vi "init_chromatic_confocal.vi"(6 "Port":u32, 7 "IP Address":u8[](array[numeric])=[192, 168, 1, 1], 9 "timeout":u32=5000 caption="Timeout", 10 "Device ID":i32 min=0 max=2, 11 "Comm Interface":enum8{"USB", "ETHERNET"}(ring)) -> (0 "error out":errorcluster {"code" format="%x"})   [LabVIEW 2020]
uses:
  Keyence CL-3000/Public/clusters/CL3IF_ETHERNET_SETTING.ctl
  Keyence CL-3000/Keyence CL-3000.lvlib
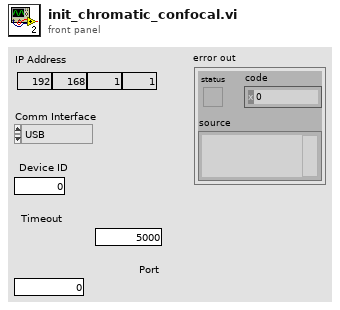
[diagram p1: front panel]
types:
  T1 = typedef "Keyence CL-3000.lvlib/CL3IF_ETHERNET_SETTING.ctl" = cluster{"IP Address":cluster{"IP1":u8, "IP2":u8, "IP3":u8, "IP4":u8}, "portNo":u32}
  T2 = cluster{"IP Address":u8, "IP Address":u8, "IP Address":u8, "IP Address":u8}
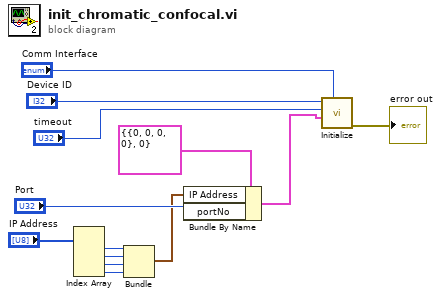
[diagram p0: block diagram]
diagram:
  n1 = Index Array(array="IP Address") -> (element #1=w4:u8, element #2=w5:u8, element #3=w6:u8, element #4=w7:u8)  [unwired: 4 in]
  n2 = Bundle("IP Address"=w4, "IP Address"=w5, "IP Address"=w6, "IP Address"=w7) -> (w8:T2)  [unwired: 1 in]
  n3 = Bundle By Name(cluster=T1 {"IP Address"={"IP1"=0, "IP2"=0, "IP3"=0, "IP4"=0}, "portNo"=0} ("ethernetSetting"), "IP Address"=w8, "portNo"="Port") -> (w12:T1)
  n4 = call "Initialize.vi"("Comm Interface"="Comm Interface", "ethernetSetting"=w12, "timeout"="timeout", "deviceId"="Device ID") -> ("error out"=→"error out":errorcluster)  [unwired: 7 in]
